vi "LSCI332 SetResistance.vi"(0 "Résistance":u16=50 caption="Résistance Chauffage", 11 "error in":errorcluster) -> (15 "error out":errorcluster)   [LabVIEW 2012]
doc: "Ce Vi envoie à l'instrument la valeur de \"Manual output\" de chauffage désiré, en %."
uses:
  <vilib>/Utility/config.llb/Write Key (I32).vi
  <vilib>/Utility/config.llb/NI_LVConfig.lvlib
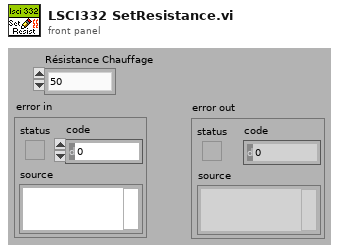
[diagram p1: front panel]
types:
  T1 = typedef "NI_LVConfig.lvlib/Config Data RefNum.ctl" = refnum<k1>
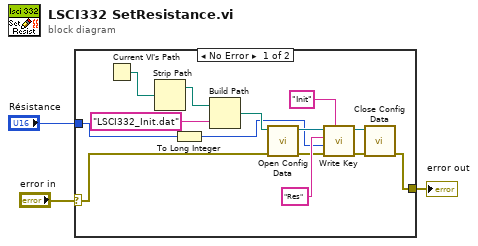
[diagram p0: block diagram]
diagram:
  n1 = case shown="No Error" "error in" {
    selector: "error in" -> [w13 w18]
    tunnel: [w7 w18] -> w3
    tunnel: "Résistance" -> [w6 _]
    frame No Error {
      n2 = Current VI's Path() -> (path=w17:path)
      n3 = Strip Path(path=w17) -> (stripped path=w16:path)  [unwired: 1 out]
      n4 = To Long Integer(number=w6) -> (32bit integer=w5:i32)
      n5 = Build Path(base path=w16, name or relative path="LSCI332_Init.dat") -> (appended path=w14:path)
      n6 = call <vilib>:"Open Config Data.vi"("error in (no error)"=w13, "configuration file path"=w14) -> ("error out"=w9:errorcluster, "refnum"=w12:T1)  [unwired: 7 in, 1 out]
      n7 = call-poly <vilib>:"Write Key.vi"("section"="Init", "error in (no error)"=w9, "value"=w5, "key"="Res", "refnum"=w12) -> ("error out"=w8:errorcluster, "refnum out"=w4:T1)  [unwired: 4 in, 1 out]
      n8 = call <vilib>:"Close Config Data.vi"("error in (no error)"=w8, "refnum"=w4) -> ("error out"=w7:errorcluster)  [unwired: 8 in, 1 out]
    }
    frame Error {
    }
  }
  "error out" <- w3
